vi "Create Temporary Directory.vi"(8 "error in":errorcluster) -> (0 "error out":errorcluster, 3 "created path":path)   [LabVIEW 2019]
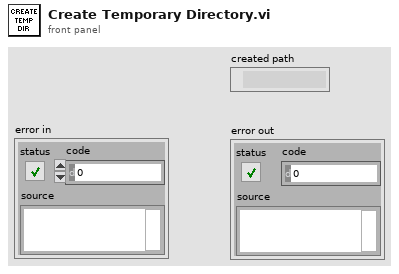
[diagram p1: front panel]
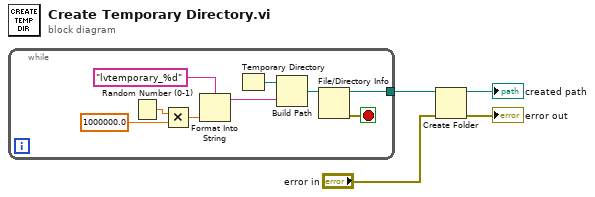
[diagram p0: block diagram]
diagram:
  n1 = while {
    tunnel: [w5] -> w4
    stop <- w6 stop-if-true
    n2 = Random Number (0-1)() -> (number: 0 to 1=w13:dbl)
    n3 = Multiply(x=w13, y=1000000.0) -> (x*y=w10:dbl)
    n4 = Format Into String(format string="lvtemporary_%d", w10) -> (resulting string=w9:string)  [unwired: 2 in, 1 out]
    n5 = Temporary Directory() -> (w8:path)
    n6 = Build Path(base path=w8, name or relative path=w9) -> (appended path=w7:path)
    n7 = File/Directory Info(path=w7) -> (path out=w5:path, error out=w6:errorcluster)  [unwired: 1 in, 5 out]
  }
  n8 = Create Folder(path (use dialog)=w4, error in="error in") -> (created path=→"created path":path, error out=→"error out":errorcluster)  [unwired: 1 in, 1 out]
